vi "cal_multilines_heights_and_widths.vi"(0 "Ring Command":string="test2:a\ntest2:bdv\ntest2:cvdvd", 1 "FP Character Width":i32=7, 5 "Strings And Values []":T1[](array[typedef])=[{"String"="AM", "Value"=0.0}, {"String"="FM", "Value"=1.0}, {"String"="ODFM", "Value"=2.0}], 7 "BD Character Width":i32=7, 9 "BD Character Height":i32=6, 11 "error in (no error)":errorcluster) -> (4 "BD Width":i32=81, 6 "BD Height":i32=27, 10 "FP Width":i32=58, 15 "error out":errorcluster)   [LabVIEW 2018]
uses:
  TypeDefinitions/ring_string_and_value.ctl
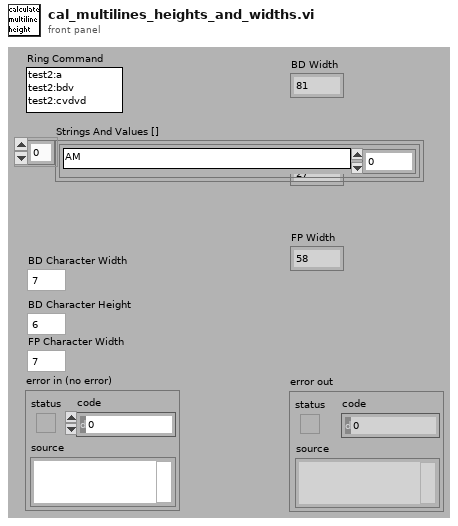
[diagram p1: front panel]
types:
  T1 = typedef "ring_string_and_value.ctl" = cluster{"String":string, "Value":dbl}
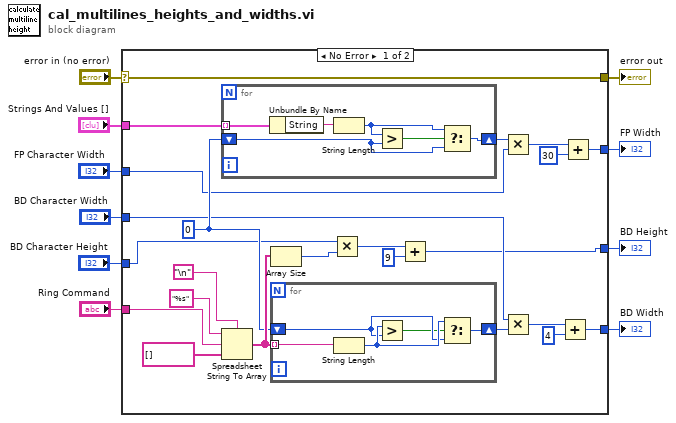
[diagram p0: block diagram]
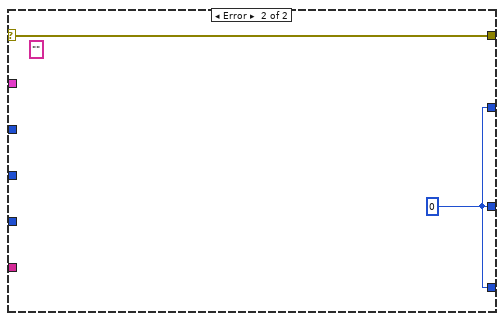
[diagram p2: hidden frame]
diagram:
  n1 = case shown="No Error" "error in (no error)" {
    selector: "error in (no error)" -> [w28 w46]
    tunnel: [w17 w45] -> w10
    tunnel: "Ring Command" -> [w30 _]
    tunnel: [w11 w45] -> w8
    tunnel: "Strings And Values []" -> [w32 _]
    tunnel: [w28 w46] -> w5
    tunnel: [w19 w45] -> w4
    tunnel: "BD Character Width" -> [w21 _]
    tunnel: "BD Character Height" -> [w20 _]
    tunnel: "FP Character Width" -> [w14 _]
    frame No Error {
      w25 = 0
      n2 = for {
        shift-right: [w41] -> w15
        shift-left: w25 -> [w42]
        tunnel: w32 -> [w40] mode=indexing
        n3 = Unbundle By Name(w40) -> ("String"=w39:string)
        n4 = String Length(string=w39) -> (length=w43:i32)
        n5 = Greater?(x=w43, y=w42) -> (0:w44:bool)
        n6 = Select(t=w43, s=w44, f=w42) -> (s? t:f=w41:i32)
      }
      n7 = Spreadsheet String To Array(delimiter (Tab)="\n", format string="%s", spreadsheet string=w30, array type (2D Dbl)=string[] []) -> (array=w26:string[])
      n8 = Array Size(array=w26) -> (size(s)=w27:i32)
      n9 = for {
        tunnel: w26 -> [w38] mode=indexing
        shift-right: [w35] -> w24
        shift-left: w25 -> [w36]
        n10 = String Length(string=w38) -> (length=w37:i32)
        n11 = Greater?(x=w37, y=w36) -> (0:w34:bool)
        n12 = Select(t=w37, s=w34, f=w36) -> (s? t:f=w35:i32)
      }
      n13 = Multiply(x=w20, y=w27) -> (x*y=w33:i32)
      n14 = Add(x=w33, y=9) -> (x+y=w17:i32)
      n15 = Multiply(x=w15, y=w14) -> (x*y=w13:i32)
      n16 = Multiply(x=w21, y=w24) -> (x*y=w22:i32)
      n17 = Add(x=w22, y=4) -> (x+y=w19:i32)
      n18 = Add(x=w13, y=30) -> (x+y=w11:i32)
    }
    frame Error {
      (unwired) ""
      w45 = 0
    }
  }
  "BD Height" <- w10
  "FP Width" <- w8
  "error out" <- w5
  "BD Width" <- w4
